vi "String to Access Type.vi"(8 "error in (no error)":errorcluster, 11 "Access Type String":string) -> (0 "error out":errorcluster, 3 "Access Type":enum32{"Read only", "Write only", "Read/write"}(ring)=enum."Read/write")   [LabVIEW 2024]
doc: "Converts a string to an access type and generates a user-defined error if the conversion fails."
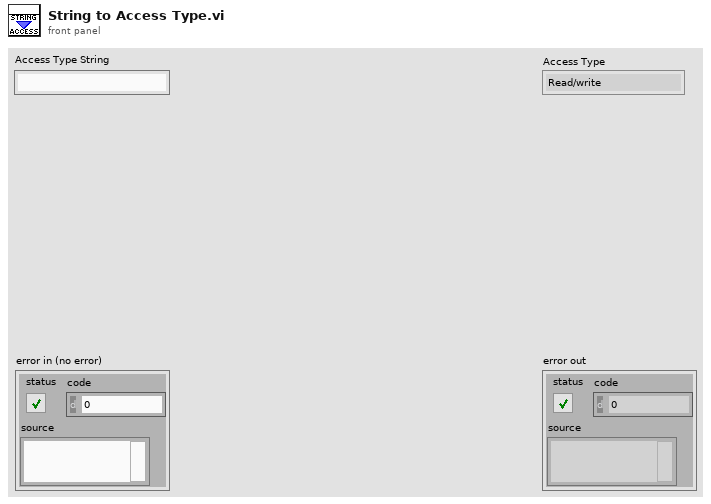
[diagram p1: front panel]
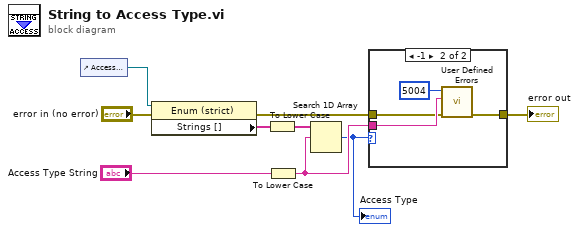
[diagram p0: block diagram]
diagram:
  n1 = control-ref of="Access Type"() -> (w6:refnum<vi>)
  n2 = property on="Property Node" class="Enum (strict)"(reference=w6, error in="error in (no error)") -> (error out=w1:errorcluster, "Strings []"=w5:string[])  [unwired: 1 out]
  n3 = To Lower Case(string=w5) -> (all lower case string=w4:string[])
  n4 = To Lower Case(string="Access Type String") -> (all lower case string=w8:string)
  n5 = Search 1D Array(1D array=w4, element=w8) -> (index of element=w3:i32)  [unwired: 1 in]
  "Access Type" <- w3
  n6 = case shown="-1" w3 {
    tunnel: w8 -> [_ w12]
    tunnel: [w10 w13] -> w7
    tunnel: w1 -> [w10 w11]
    frame Default {
    }
    frame -1 {
      n7 = call "User Defined Errors.vi"("error in (no error)"=w11, "Parameter 1"=w12, "Error Code (0)"=5004 ("error code (0)")) -> ("error out"=w13:errorcluster)  [unwired: 8 in]
    }
  }
  "error out" <- w7
